vi "NodeFormula.vi"() -> ()   [LabVIEW 2015]
panel:
  out "output variable 2":dbl
  out "x*y 2":dbl
  out "x*y":dbl
  out "output variable":dbl
  in  "Nivel":dbl
  in  "Presion":dbl
  in  "Temperatura":dbl
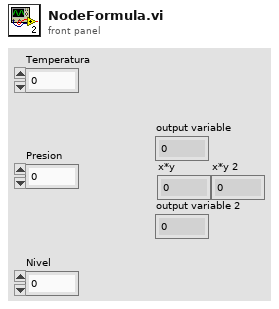
[diagram p1: front panel]
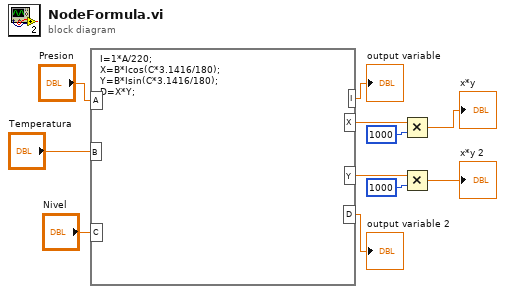
[diagram p0: block diagram]
diagram:
  n1 = formula code="I=1*A/220;\nX=B*Icos(C*3.1416/180);\nY=B*Isin(C*3.1416/180);\nD=X*Y;"("A"="Presion", "B"="Temperatura", "C"="Nivel") -> ("I"=→"output variable":dbl, "X"=w7:dbl, "Y"=w3:dbl, "D"=→"output variable 2":dbl)
  n2 = Multiply(x=w7, y=1000) -> (x*y=→"x*y":dbl)
  n3 = Multiply(x=w3, y=1000) -> (x*y=→"x*y 2":dbl)
